vi "_Obtain CSMQ.vi"(8 "Error in":errorcluster caption="Error in (no error)", 9 "create if not found? (T)":bool=TRUE, 11 "Name(\"\" to use uuid) in":string) -> (0 "Error out":errorcluster, 1 "Create(T)/Cached(F)":bool, 3 "CSM-Obj":T1, 4 "Name":string)   [LabVIEW 2014, in "Communicable State Machine.lvlib"]
uses:
  Communicable State Machine.lvlib
  _CSMObj.ctl
  Priority Queue/Priority Queue.lvclass
  Typedef/_CSM_MODE.ctl
  Typedef/_CSM Status Change Event Data.ctl
  Priority Queue/Priority Queue.lvclass/Priority Queue.ctl
  _CSMQFGVOPER.ctl
  FGV-BroadcastRegistry/global-CSMQ FGV Change Flag.vi
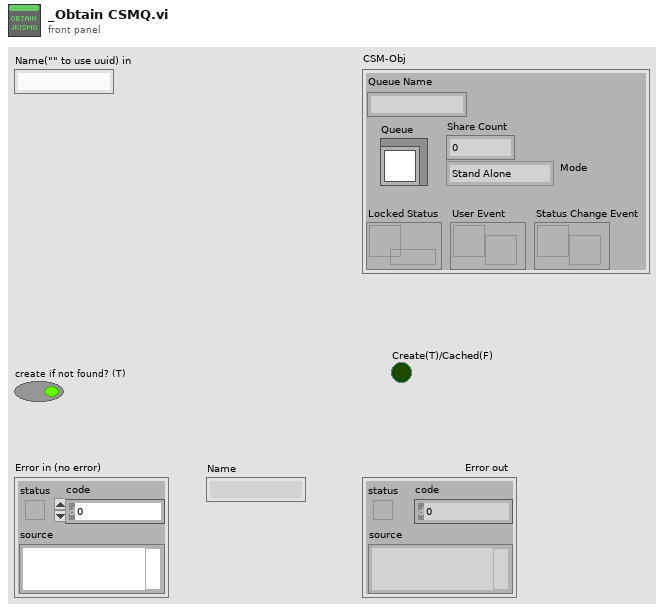
[diagram p1: front panel]
types:
  T1 = typedef "Communicable State Machine.lvlib/_CSMObj.ctl" = cluster{"Queue Name":string, "Mode":T2, "Share Count":i32, "Queue":refnum<class "Priority Queue.lvclass">, "Locked Status":refnum<data-value>, "User Event":refnum<user-event>, "Status Change Event":refnum<user-event>}
  T2 = typedef "Communicable State Machine.lvlib/_CSM_MODE.ctl" = enum16{"Stand Alone", "CSM", "Action Worker"}
  T3 = typedef "Communicable State Machine.lvlib/_CSMQFGVOPER.ctl" = enum16{"Get By Name", "List", "Check If Name Exists", "Release", "Module Status", "Create Status Event Handler", "Destroy Status Event Handler"}
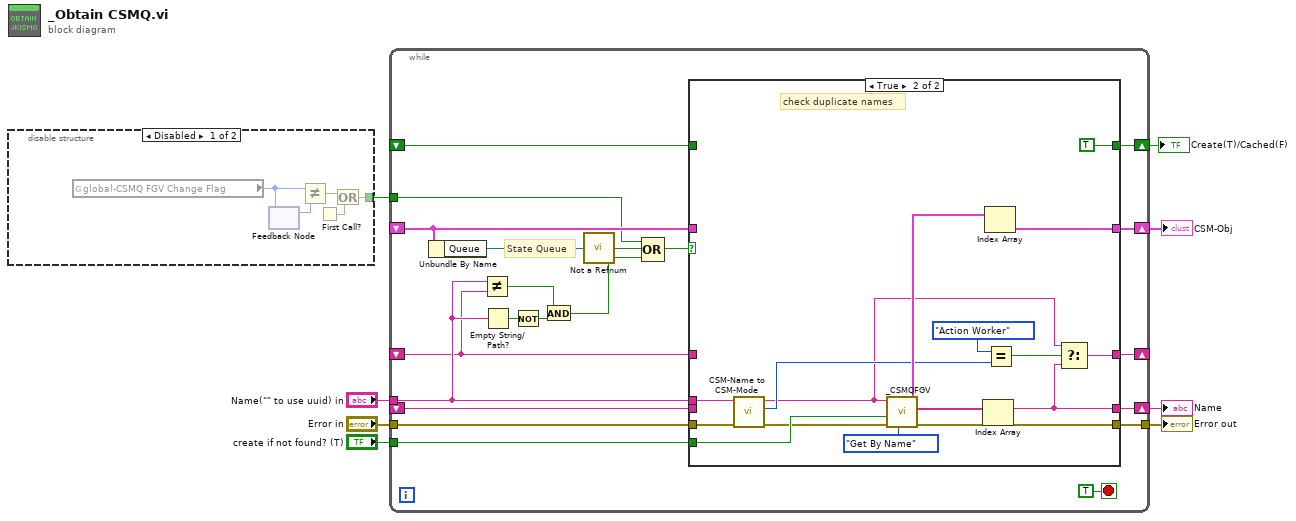
[diagram p0: block diagram]
diagram:
  n1 = disable-structure shown="Disabled" {
    disable-tunnel: [w9 _] -> w2
    frame Disabled {
      n2 = global read "global-CSMQ FGV Change Flag.vi" "global-CSMQ FGV Change Flag"() -> (w10:u32)
      n3 = feedback #1() -> (w11:u32)  [unwired: 1 in]
      n4 = feedback-in #1(w10) -> ()
      n5 = Not Equal?(x=w10, y=w11) -> (x != y?=w13:bool)
      n6 = First Call?() -> (First Call?: T/F=w12:bool)
      n7 = Or(x=w13, y=w12) -> (x .or. y?=w9:bool)
    }
    frame Enabled {
    }
  }
  n8 = while {
    shift-right: [w32] -> w8
    shift-left: _ -> [w27]
    shift-right: [w31] -> w3
    shift-left: _ -> [w23]
    tunnel: "create if not found? (T)" -> [w30]
    tunnel: "Error in" -> [w29]
    tunnel: [w28] -> w5
    tunnel: "Name(\"\" to use uuid) in" -> [w24]
    shift-right: [w18] -> _
    shift-left: _ -> [w17]
    tunnel: w2 -> [w16]
    shift-right: [w14] -> w1
    shift-left: _ -> [w15]
    stop <- TRUE stop-if-true
    # "State Queue"
    n9 = Unbundle By Name(w23) -> ("Queue"=w22:refnum<class "Priority Queue.lvclass">)
    n10 = Not Equal?(x=w24, y=w17) -> (x != y?=w21:bool)
    n11 = Empty String/Path?(string/path=w24) -> (empty?=w20:bool)
    n12 = Not(x=w20) -> (.not. x?=w19:bool)
    n13 = And(x=w21, y=w19) -> (x .and. y?=w25:bool)
    n14 = call "Not a Refnum.vi"("Priority Queue.lvclass"=w22) -> ("NaN/Path/Refnum?"=w33:bool)  [unwired: 4 in]
    n15 = Compound Arithmetic op=OR(w16, w33, w25) -> (w26:bool)
    n16 = case shown="True" w26 {
      tunnel: w27 -> [w38 _]
      tunnel: [w38 w43] -> w32
      tunnel: [w37 w48] -> w31
      tunnel: w23 -> [w37 _]
      tunnel: w30 -> [_ w49]
      tunnel: w29 -> [w36 w39]
      tunnel: [w36 w50] -> w28
      tunnel: w24 -> [_ w40]
      tunnel: [w35 w42] -> w18
      tunnel: w17 -> [w35 _]
      tunnel: w15 -> [_ _]
      tunnel: [_ TRUE] -> w14
      frame False {
      }
      frame True {
        # "check duplicate names"
        n17 = call "CSM-Name to CSM-Mode.vi"("String"=w40) -> ("CSM Mode"=w47:T2, "String(dup)"=w44:string)  [unwired: 8 in, 1 out]
        n18 = call "_CSMQFGV.vi"("Operation"=_CSMQFGVOPER."Get By Name", "Error in"=w39, "create if not found? (T)"=w49, "Name(\"\" to use uuid) in"=w44) -> ("Error out"=w50:errorcluster, "Name"=w51:string[], "Array"=w53:T1[])  [unwired: 4 in, 1 out]
        n19 = Index Array(array=w51) -> (element=w43:string)  [unwired: 1 in]
        n20 = Index Array(array=w53) -> (element=w48:T1)  [unwired: 1 in]
        n21 = Equal?(x=_CSM_MODE."Action Worker", y=w47) -> (x = y?=w45:bool)
        n22 = Select(t=w44, s=w45, f=w43) -> (s? t:f=w42:string)
      }
    }
  }
  "Error out" <- w5
  "CSM-Obj" <- w3
  "Name" <- w8
  "Create(T)/Cached(F)" <- w1
